vi "Split.vi"(6 "Groups":string[][](array[string]), 8 "error in (no error)":errorcluster caption="entrée d'erreur (pas d'erreur)", 9 "y":string[][](array[string]), 10 "X":string[][](array[string]), 11 "LeaveOneGroupOut.lvclass":refnum<class "LeaveOneGroupOut.lvclass">) -> (0 "error out":errorcluster caption="sortie d'erreur", 2 "Split":T1(array[cluster]), 3 "LeaveOneGroupOut.lvclass":refnum<class "LeaveOneGroupOut.lvclass">)   [LabVIEW 2020, in "LeaveOneGroupOut.lvclass"]
doc: "Return : \n\n- train : ndarray\n The training set indices for that split.\n\n- test : ndarray\n The testing set indices for that split."
uses:
  LeaveOneGroupOut.lvclass
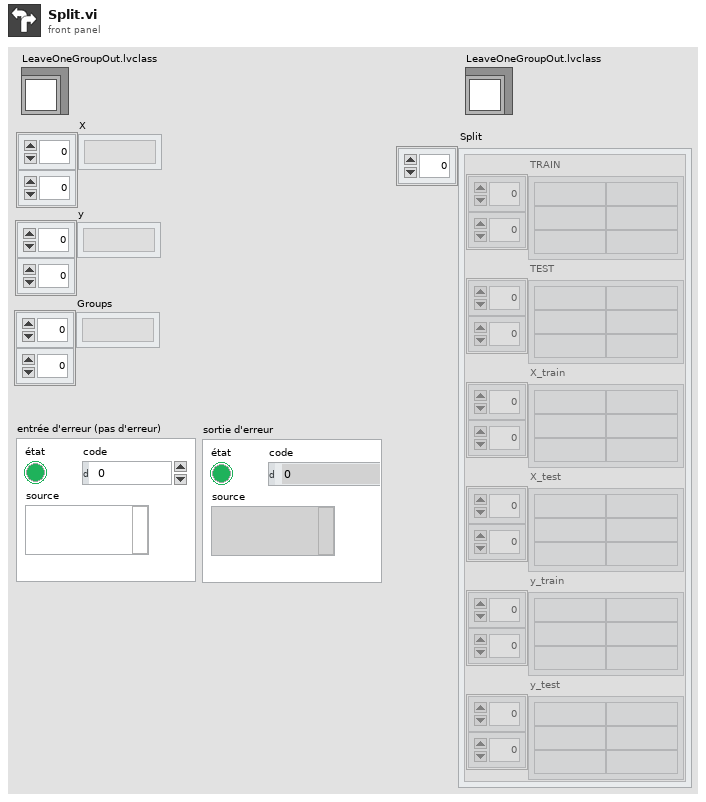
[diagram p1: front panel]
types:
  T1 = cluster{"TRAIN":string[][], "TEST":string[][], "X_train":string[][], "X_test":string[][], "y_train":string[][], "y_test":string[][]}[]
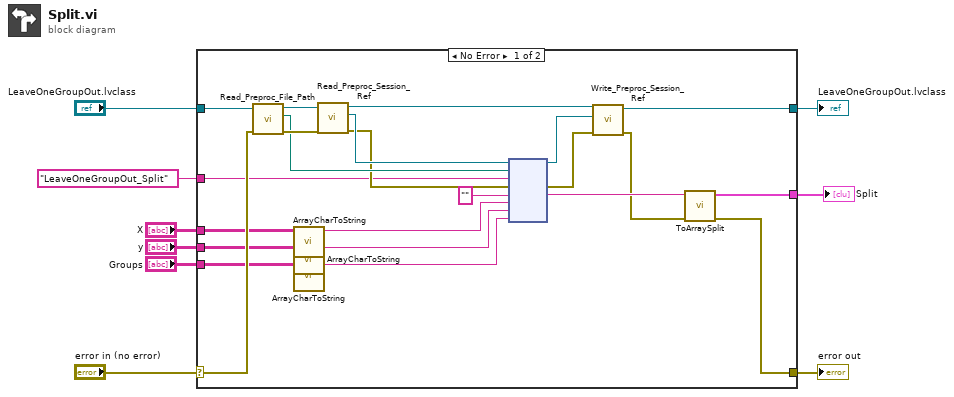
[diagram p0: block diagram]
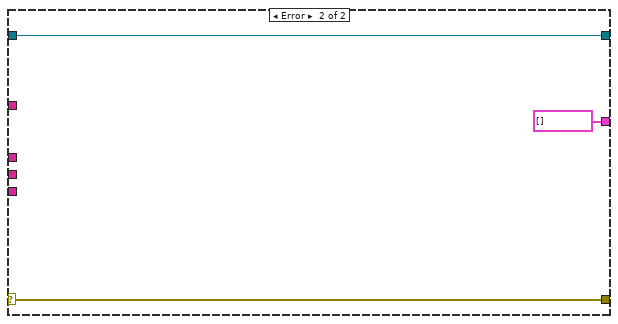
[diagram p2: hidden frame]
diagram:
  n1 = case shown="No Error" "error in (no error)" {
    selector: "error in (no error)" -> [w23 w35]
    tunnel: [w11 w35] -> w8
    tunnel: [w14 w34] -> w6
    tunnel: "LeaveOneGroupOut.lvclass" -> [w21 w34]
    tunnel: "LeaveOneGroupOut_Split" -> [w22 _]
    tunnel: "X" -> [w20 _]
    tunnel: "y" -> [w19 _]
    tunnel: "Groups" -> [w18 _]
    tunnel: [w10 T1 [] ("Split")] -> w1
    frame No Error {
      n2 = call-dynamic "Read_Preproc_File_Path.vi"("error in (no error)"=w23, "Python in"=w21) -> ("error out"=w31:errorcluster, "File_Path"=w30:path, "Python out"=w32:refnum<class "LeaveOneGroupOut.lvclass">)  [unwired: 7 in]
      n3 = call "ArrayCharToString.vi"("TAB"=w20) -> ("Instruction"=w17:string)  [unwired: 10 in]
      n4 = call "ArrayCharToString.vi"("TAB"=w19) -> ("Instruction"=w16:string)  [unwired: 10 in]
      n5 = call "ArrayCharToString.vi"("TAB"=w18) -> ("Instruction"=w15:string)  [unwired: 10 in]
      n6 = call-dynamic "Read_Preproc_Session_Ref.vi"("error in (no error)"=w31, "Python in"=w32) -> ("error out"=w28:errorcluster, "Session_ref"=w29:refnum<k35>, "Python out"=w27:refnum<class "LeaveOneGroupOut.lvclass">)  [unwired: 7 in]
      n7 = node(w29, w30, w22, w28, "", w17, w16, w15) -> (w25:refnum<k35>, w26:errorcluster, w13:string)  [unwired: 3 in, 2 out]
      n8 = call-dynamic "Write_Preproc_Session_Ref.vi"("error in (no error)"=w26, "Session_ref"=w25, "Python in"=w27) -> ("error out"=w12:errorcluster, "Python out"=w14:refnum<class "LeaveOneGroupOut.lvclass">)  [unwired: 7 in]
      n9 = call "ToArraySplit.vi"("sortie d'erreur"=w12, "Return value"=w13) -> ("sortie d'erreur"=w11:errorcluster, "Split"=w10:T1)  [unwired: 8 in]
    }
    frame Error {
    }
  }
  "error out" <- w8
  "LeaveOneGroupOut.lvclass" <- w6
  "Split" <- w1
